vi "TRAPBALL.vi"   [LabVIEW 2016, in "Test2.lvrbt"]
uses:
  Test2.lvrbt
  <vilib>/NXT/Block Support/NXT_InputPort.ctl
  <vilib>/NXT/Hardware/Plugins/Tetrix DC Motor/TetrixDCMotorAddress.ctl
  <vilib>/NXT/Hardware/Plugins/Tetrix 180 deg Servo/Tetrix180ServoAddress.ctl
  <vilib>/NXT/NXTIO Xnodes/NXTIONodeSubVIs/TETRIX IO Move Servos.vi
  <vilib>/NXT/Dual Mode Library/Waits/Wait_Num.vi
  <vilib>/NXT/NXTIO Xnodes/NXTIONodeSubVIs/TETRIX IO Move DC Motors.vi
  <vilib>/NXT/Dual Mode Library/Waits/Wait_EV3_Ultrasonic_Centimeters_Further.vi
  <vilib>/NXT/NXTIO Xnodes/NXTIONodeSubVIs/TETRIX IO Stop DC Motors.vi
  <vilib>/NXT/NXTIO Xnodes/AddressXNode/NXTIOAddress.xnode
  <vilib>/NXT/Subs/LVHSConnector.ctl
  <vilib>/NXT/NXTIO Xnodes/NXTIOXNode/NXTIO.xnode
  <vilib>/NXT/LegoClasses/BrickReference/BrickReference.lvclass
types:
  T1 = typedef "NXT_InputPort.ctl" = u32
  T2 = typedef "Tetrix180ServoAddress.ctl" = i32
  T3 = cluster{"Tetrix180Servo":T2, "Tetrix180Servo":T2, "Tetrix180Servo":T2, "Tetrix180Servo":T2, "Tetrix180Servo":T2, "Tetrix180Servo":T2}
  T4 = typedef "LVHSConnector.ctl" = refnum<class "BrickReference.lvclass">
  T5 = typedef "TetrixDCMotorAddress.ctl" = i32
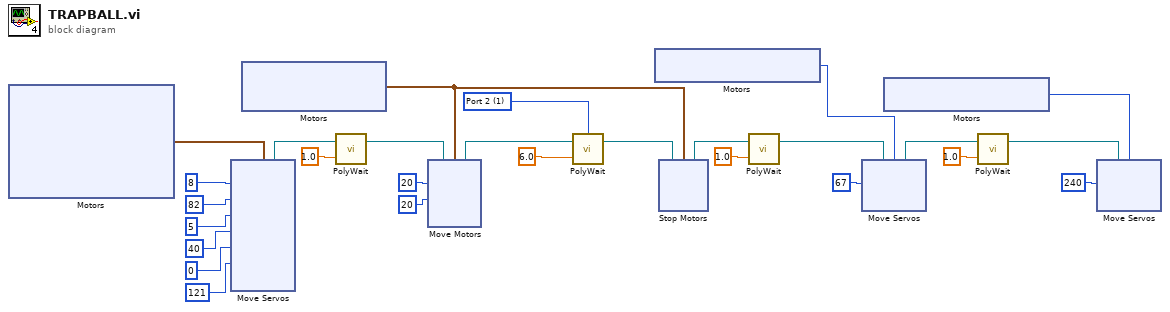
[diagram p0: block diagram]
diagram:
  w24 = T1 1 items=["Port 1", "Port 2", "Port 3", "Port 4"] ("Port (Port 1)")
  n1 = xnode "Motors"() -> ("Motor"=w20:T3)
  n2 = xnode "Move Servos"("Position 6"=u8 121, "Position 5"=u8 0, "Position 4"=u8 40, "Position 3"=u8 5, "Position 2"=u8 82, "Position 1"=u8 8, "Motors"=w20) -> ("NXT/EV3"=w13:T4)  [unwired: 1 in]
  n3 = xnode "Motors"() -> ("Motor"=w21:cluster{"TetrixDCMotor":T5, "TetrixDCMotor":T5})
  n4 = call-poly <vilib>:"PolyWait.vi"("Time (1 sec)"=sgl 1.0, "NXT/EV3"=w13) -> ("NXT/EV3"=w11:T4)  [unwired: 2 in]
  n5 = xnode "Move Motors"("Power/Speed 2"=i8 20, "Power/Speed 1"=i8 20, "Motors"=w21, "NXT/EV3"=w11) -> ("NXT/EV3"=w27:T4)
  n6 = call-poly <vilib>:"PolyWait.vi"("Centimeters (50)"=sgl 6.0, "NXT/EV3"=w27, "Port (Port 1)"=w24) -> ("NXT/EV3"=w25:T4)  [unwired: 1 in]
  n7 = xnode "Motors"() -> ("Motor"=w8:T2)
  n8 = xnode "Stop Motors"("Motors"=w21, "NXT/EV3"=w25) -> ("NXT/EV3"=w1:T4)
  n9 = call-poly <vilib>:"PolyWait.vi"("Time (1 sec)"=sgl 1.0, "NXT/EV3"=w1) -> ("NXT/EV3"=w7:T4)  [unwired: 2 in]
  n10 = xnode "Move Servos"("Position 1"=u8 67, "Motors"=w8, "NXT/EV3"=w7) -> ("NXT/EV3"=w5:T4)
  n11 = xnode "Motors"() -> ("Motor"=w3:T2)
  n12 = call-poly <vilib>:"PolyWait.vi"("Time (1 sec)"=sgl 1.0, "NXT/EV3"=w5) -> ("NXT/EV3"=w2:T4)  [unwired: 2 in]
  n13 = xnode "Move Servos"("Position 1"=u8 240, "Motors"=w3, "NXT/EV3"=w2) -> ()  [unwired: 1 out]
